vi "Take Reading.vi"(2 "error in (no error)":errorcluster, 3 "Obstacle Boundries":dbl[][](array[numeric]), 4 "Car.lvclass":refnum<class "Car.lvclass">, 5 "SonarSensor.lvclass":refnum<class "SonarSensor.lvclass">) -> (0 "error out":errorcluster, 1 "Distance Read":dbl)   [LabVIEW 2015, in "SonarSensor.lvclass"]
uses:
  SonarSensor.lvclass
  Car.lvclass
  Sensor.lvclass
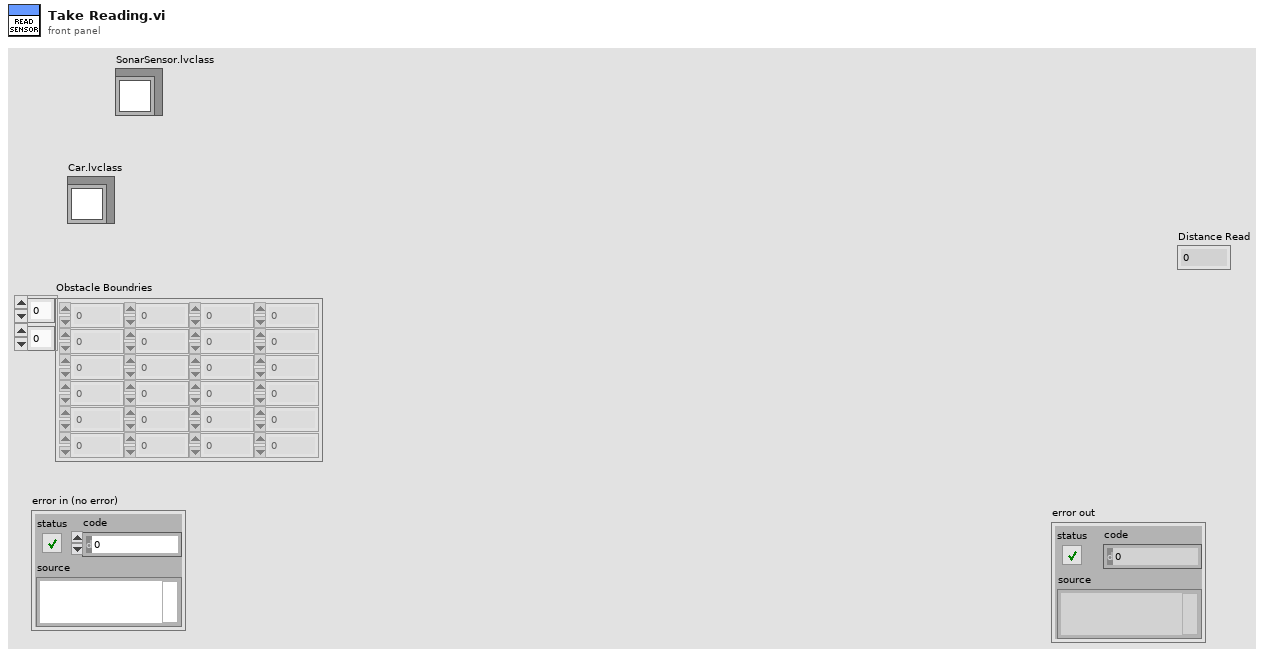
[diagram p1: front panel]
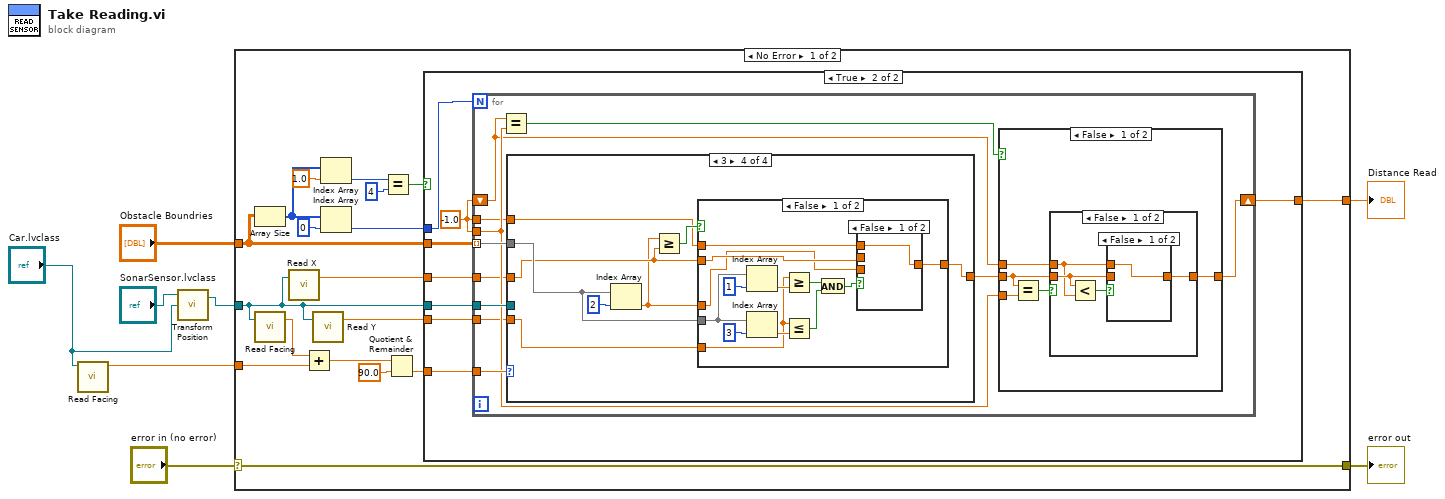
[diagram p0: block diagram]
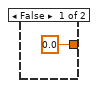
[diagram p2: hidden frame]
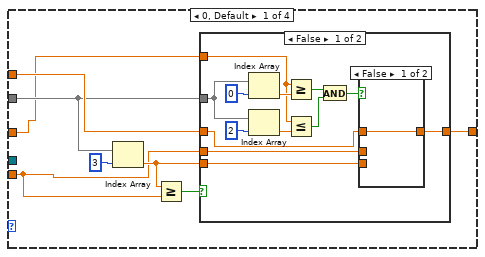
[diagram p6: hidden frame]
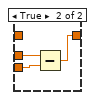
[diagram p7: hidden frame]
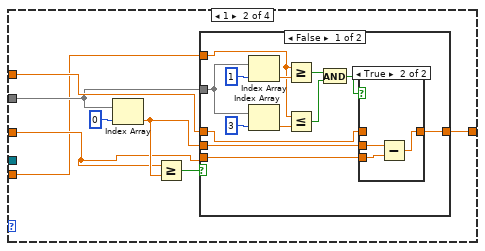
[diagram p9: hidden frame]
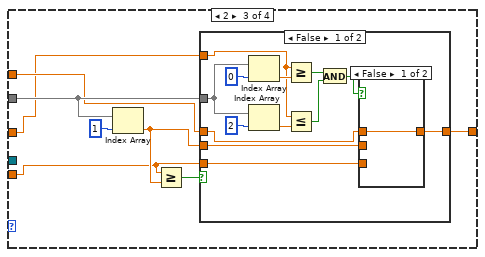
[diagram p12: hidden frame]
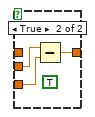
[diagram p13: hidden frame]
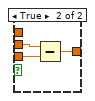
[diagram p15: hidden frame]
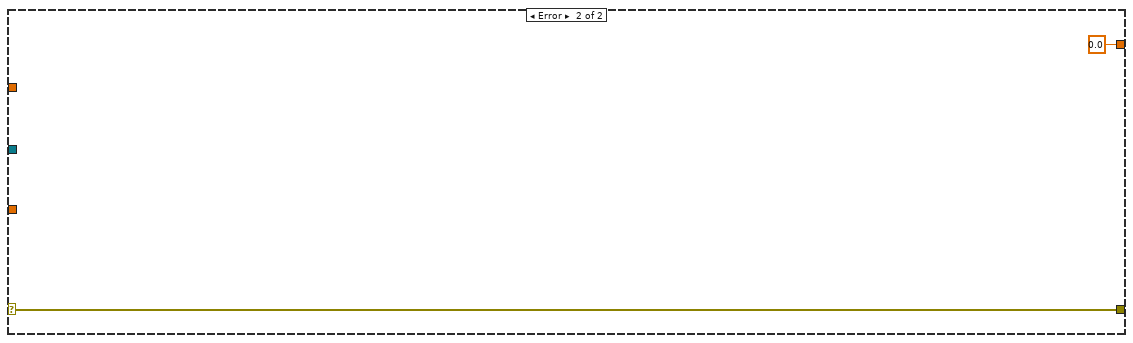
[diagram p17: hidden frame]
diagram:
  n1 = call "Read Facing.vi"("Car.lvclass"="Car.lvclass") -> ("Facing"=w4:dbl)  [unwired: 9 in, 1 out]
  n2 = call "Transform Position.vi"("Car.lvclass"="Car.lvclass", "Sensor.lvclass"="SonarSensor.lvclass") -> ("Sensor.lvclass 2"=w1:refnum<class "SonarSensor.lvclass">)  [unwired: 1 in, 1 out]
  n3 = case shown="No Error" "error in (no error)" {
    selector: "error in (no error)" -> [w12 w165]
    tunnel: [w12 w165] -> w7
    tunnel: [w23 0.0] -> w6
    tunnel: "Obstacle Boundries" -> [w16 _]
    tunnel: w1 -> [w10 _]
    tunnel: w4 -> [w13 _]
    frame No Error {
      n4 = Array Size(array=w16) -> (size(s)=w20:i32[])
      n5 = call "Read Facing.vi"("Sensor.lvclass"=w10) -> ("Facing"=w14:dbl)  [unwired: 1 in, 1 out]
      n6 = call "Read X.vi"("Sensor.lvclass"=w10) -> ("X"=w11:dbl)  [unwired: 1 in, 1 out]
      n7 = Add(x=w14, y=w13) -> (x+y=w15:dbl)
      n8 = call "Read Y.vi"("Sensor.lvclass"=w10) -> ("Y"=w9:dbl)  [unwired: 1 in, 1 out]
      n9 = Index Array(array=w20, index=1.0) -> (element=w21:i32)
      n10 = Index Array(array=w20, index=0) -> (element=w18:i32)
      n11 = Equal?(x=w21, y=4) -> (x = y?=w24:bool)
      n12 = Quotient & Remainder(x=w15, y=90.0) -> (floor(x/y)=w17:dbl)  [unwired: 1 out]
      n13 = case shown="True" w24 {
        tunnel: [0.0 w31] -> w23
        tunnel: w18 -> [_ w35]
        tunnel: w17 -> [_ w34]
        tunnel: w16 -> [_ w33]
        tunnel: w10 -> [_ w32]
        tunnel: w11 -> [_ w29]
        tunnel: w9 -> [_ w28]
        frame False {
        }
        frame True {
          w30 = -1.0
          n14 = for {
            N: w35 -> [_]
            tunnel: w34 -> [w46]
            tunnel: w33 -> [w44] mode=indexing
            tunnel: w32 -> [w45]
            shift-right: [w42] -> w31
            shift-left: w30 -> [w39]
            tunnel: w30 -> [w40]
            tunnel: w30 -> [w38]
            tunnel: w29 -> [w37]
            tunnel: w28 -> [w36]
            n15 = Equal?(x=w39, y=w40) -> (x = y?=w43:bool)
            n16 = case shown="3" w46 {
              tunnel: w44 -> [w63 w89 w117 w141]
              tunnel: w45 -> [_ _ _ _]
              tunnel: [w65 w91 w115 w143] -> w41
              tunnel: w38 -> [w64 w90 w114 w142]
              tunnel: w37 -> [w60 w87 w112 w140]
              tunnel: w36 -> [w61 w86 w113 w138]
              frame 0, Default {
                n17 = Index Array(array=w63, index=3) -> (element=w62:dbl)
                n18 = Greater Or Equal?(x=w62, y=w61) -> (x >= y?=w66:bool)
                n19 = case shown="False" w66 {
                  tunnel: [w71 w85] -> w65
                  tunnel: w64 -> [w68 w85]
                  tunnel: w63 -> [w74 _]
                  tunnel: w60 -> [w73 _]
                  tunnel: w61 -> [w70 _]
                  tunnel: w62 -> [w69 _]
                  frame False {
                    n20 = Index Array(array=w74, index=0) -> (element=w78:dbl)
                    n21 = Index Array(array=w74, index=2) -> (element=w77:dbl)
                    n22 = Greater Or Equal?(x=w73, y=w78) -> (x >= y?=w76:bool)
                    n23 = Less Or Equal?(x=w73, y=w77) -> (x <= y?=w75:bool)
                    n24 = And(x=w76, y=w75) -> (x .and. y?=w72:bool)
                    n25 = case shown="False" w72 {
                      tunnel: [w81 w84] -> w71
                      tunnel: w70 -> [_ w83]
                      tunnel: w69 -> [_ w82]
                      tunnel: w68 -> [w81 _]
                      frame False {
                      }
                      frame True {
                        n26 = Subtract(x=w83, y=w82) -> (x-y=w84:dbl)
                      }
                    }
                  }
                  frame True {
                  }
                }
              }
              frame 1 {
                n27 = Index Array(array=w89, index=0) -> (element=w88:dbl)
                n28 = Greater Or Equal?(x=w87, y=w88) -> (x >= y?=w92:bool)
                n29 = case shown="False" w92 {
                  tunnel: [w95 w111] -> w91
                  tunnel: w90 -> [w94 w111]
                  tunnel: w89 -> [w100 _]
                  tunnel: w86 -> [w99 _]
                  tunnel: w88 -> [w97 _]
                  tunnel: w87 -> [w96 _]
                  frame False {
                    n30 = Index Array(array=w100, index=1) -> (element=w103:dbl)
                    n31 = Index Array(array=w100, index=3) -> (element=w104:dbl)
                    n32 = Greater Or Equal?(x=w99, y=w103) -> (x >= y?=w106:bool)
                    n33 = Less Or Equal?(x=w99, y=w104) -> (x <= y?=w105:bool)
                    n34 = And(x=w106, y=w105) -> (x .and. y?=w98:bool)
                    n35 = case shown="True" w98 {
                      tunnel: w97 -> [_ w110]
                      tunnel: w96 -> [_ w109]
                      tunnel: [w107 w108] -> w95
                      tunnel: w94 -> [w107 _]
                      frame False {
                      }
                      frame True {
                        n36 = Subtract(x=w110, y=w109) -> (x-y=w108:dbl)
                      }
                    }
                  }
                  frame True {
                  }
                }
              }
              frame 2 {
                n37 = Index Array(array=w117, index=1) -> (element=w116:dbl)
                n38 = Greater Or Equal?(x=w113, y=w116) -> (x >= y?=w118:bool)
                n39 = case shown="False" w118 {
                  tunnel: w117 -> [w132 _]
                  tunnel: w112 -> [w127 _]
                  tunnel: w116 -> [w123 _]
                  tunnel: w113 -> [w122 _]
                  tunnel: [w121 w137] -> w115
                  tunnel: w114 -> [w120 w137]
                  frame False {
                    n40 = Index Array(array=w132, index=0) -> (element=w129:dbl)
                    n41 = Index Array(array=w132, index=2) -> (element=w128:dbl)
                    n42 = Greater Or Equal?(x=w127, y=w129) -> (x >= y?=w126:bool)
                    n43 = Less Or Equal?(x=w127, y=w128) -> (x <= y?=w125:bool)
                    n44 = And(x=w126, y=w125) -> (x .and. y?=w124:bool)
                    n45 = case shown="False" w124 {
                      tunnel: w123 -> [_ w136]
                      tunnel: w122 -> [_ w135]
                      tunnel: [w133 w134] -> w121
                      tunnel: w120 -> [w133 _]
                      frame False {
                      }
                      frame True {
                        (unwired) TRUE
                        n46 = Subtract(x=w136, y=w135) -> (x-y=w134:dbl)
                      }
                    }
                  }
                  frame True {
                  }
                }
              }
              frame 3 {
                n47 = Index Array(array=w141, index=2) -> (element=w139:dbl)
                n48 = Greater Or Equal?(x=w139, y=w140) -> (x >= y?=w144:bool)
                n49 = case shown="False" w144 {
                  tunnel: [w148 w163] -> w143
                  tunnel: w142 -> [w147 w163]
                  tunnel: w141 -> [w158 _]
                  tunnel: w140 -> [w150 _]
                  tunnel: w139 -> [w149 _]
                  tunnel: w138 -> [w146 _]
                  frame False {
                    n50 = Index Array(array=w158, index=1) -> (element=w155:dbl)
                    n51 = Index Array(array=w158, index=3) -> (element=w154:dbl)
                    n52 = Greater Or Equal?(x=w146, y=w155) -> (x >= y?=w152:bool)
                    n53 = Less Or Equal?(x=w146, y=w154) -> (x <= y?=w153:bool)
                    n54 = And(x=w152, y=w153) -> (x .and. y?=w151:bool)
                    n55 = case shown="False" w151 {
                      tunnel: w150 -> [_ w162]
                      tunnel: w149 -> [_ w161]
                      tunnel: [w159 w160] -> w148
                      tunnel: w147 -> [w159 _]
                      frame False {
                      }
                      frame True {
                        n56 = Subtract(x=w162, y=w161) -> (x-y=w160:dbl)
                      }
                    }
                  }
                  frame True {
                  }
                }
              }
            }
            n57 = case shown="False" w43 {
              tunnel: [w49 w59] -> w42
              tunnel: w41 -> [w47 w59]
              tunnel: w40 -> [w51 _]
              tunnel: w39 -> [w48 _]
              frame False {
                n58 = Equal?(x=w47, y=w51) -> (x = y?=w50:bool)
                n59 = case shown="False" w50 {
                  tunnel: [w53 w58] -> w49
                  tunnel: w48 -> [w52 w58]
                  tunnel: w47 -> [w54 _]
                  frame False {
                    n60 = Less?(x=w54, y=w52) -> (x < y?=w55:bool)
                    n61 = case shown="False" w55 {
                      tunnel: w54 -> [_ w57]
                      tunnel: [w56 w57] -> w53
                      tunnel: w52 -> [w56 _]
                      frame False {
                      }
                      frame True {
                      }
                    }
                  }
                  frame True {
                  }
                }
              }
              frame True {
              }
            }
          }
        }
      }
    }
    frame Error {
    }
  }
  "error out" <- w7
  "Distance Read" <- w6
